vi "LIST FILE NAMES.vi"(8 "error in (no error)":errorcluster) -> (0 "error out":errorcluster, 3 "filenames":string[](array[string]))   [LabVIEW 2025]
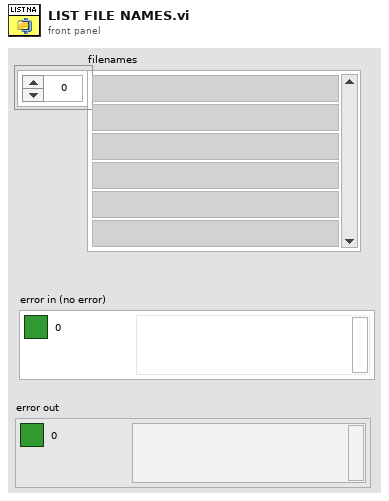
[diagram p1: front panel]
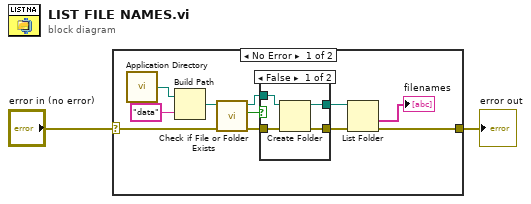
[diagram p0: block diagram]
diagram:
  n1 = case shown="No Error" "error in (no error)" {
    selector: "error in (no error)" -> [w4 _]
    tunnel: [w5 _] -> w1
    frame No Error {
      n2 = call <vilib>:"Application Directory.vi"() -> ("Application Directory"=w7:path)
      n3 = Build Path(base path=w7, name or relative path="data") -> (appended path=w6:path)
      n4 = call <vilib>:"Check if File or Folder Exists.vi"("error in (no error)"=w4, "path"=w6) -> ("error out"=w13:errorcluster, "file or folder exists?"=w11:bool, "dup path"=w12:path)  [unwired: 7 in]
      n5 = case shown="False" w11 {
        tunnel: w12 -> [w17 w18]
        tunnel: w13 -> [w16 w19]
        tunnel: [w15 w19] -> w9
        tunnel: [w14 w18] -> w10
        frame False {
          n6 = Create Folder(path (use dialog)=w17, error in=w16) -> (created path=w14:path, error out=w15:errorcluster)  [unwired: 1 in, 1 out]
        }
        frame True {
        }
      }
      n7 = List Folder(path=w10, error in=w9) -> (folder names=→"filenames":string[], error out=w5:errorcluster)  [unwired: 2 in, 2 out]
    }
    frame Error {
    }
  }
  "error out" <- w1
